vi "ErrorCheckHWI.vi"(8 "error in (no error)":errorcluster, 11 "LTA-HS in":refnum<class "LTA-HS.lvclass">) -> (0 "error out":errorcluster, 3 "LTA-HS out":refnum<class "LTA-HS.lvclass">)   [LabVIEW 2013, in "LTA-HS.lvclass"]
uses:
  LTA-HS.lvclass
  Device/Device.lvclass
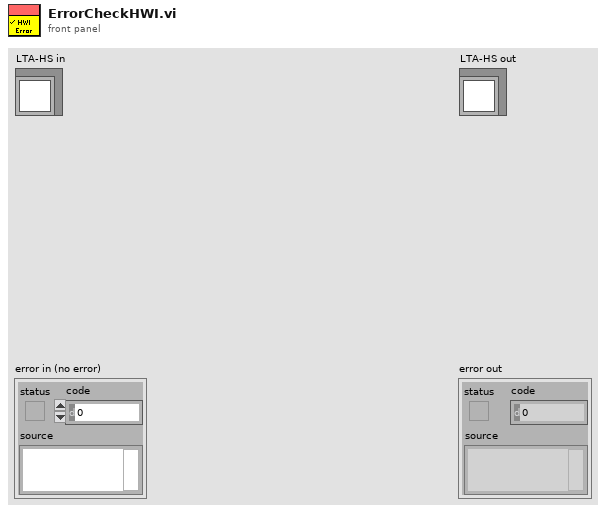
[diagram p1: front panel]
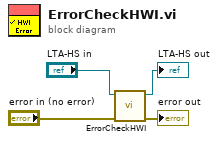
[diagram p0: block diagram]
diagram:
  n1 = call-parent "ErrorCheckHWI.vi"("error in (no error)"="error in (no error)", "Device in"="LTA-HS in") -> ("error out"=→"error out":errorcluster, "Device out"=→"LTA-HS out":refnum<class "LTA-HS.lvclass">)  [unwired: 8 in]
